vi "Single Channel_stepper.vi"(4 "B":bool, 5 "A":bool, 6 "DIR":bool, 7 "Period (Ticks)":u32=2000, 8 "STBY":bool, 9 "ENA":bool, 10 "Duty":fxp<+,32,0>, 11 "I/O Channel":T1={"Encoder C"="ConnectorA/DIO13", "Encoder B"="ConnectorA/DIO12", "Encoder A"="ConnectorA/DIO11", "PWM"="ConnectorA/DIO10", "DIR"="ConnectorA/DIO9", "STBY"="ConnectorA/DIO8", "ENA"="ConnectorA/DIO7"}) -> (1 "C":bool)   [LabVIEW 2018]
uses:
  <vilib>/rvi/eio/common/nirviEmuTemplateMethod_errors.vi
  <vilib>/eio/EIONode/EIONode.xnode
  jmslib.lvlib
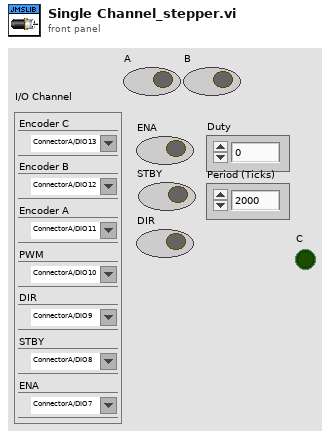
[diagram p1: front panel]
types:
  T1 = cluster{"Encoder C":refnum<k21>, "Encoder B":refnum<k21>, "Encoder A":refnum<k21>, "PWM":refnum<k21>, "DIR":refnum<k21>, "STBY":refnum<k21>, "ENA":refnum<k21>}
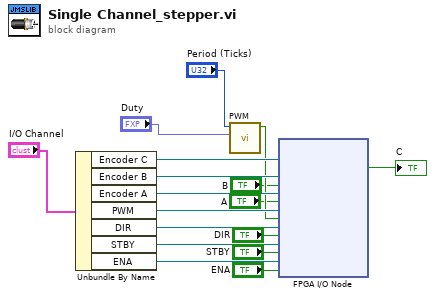
[diagram p0: block diagram]
diagram:
  n1 = Unbundle By Name("I/O Channel") -> ("Encoder C"=w16:refnum<k21>, "Encoder B"=w15:refnum<k21>, "Encoder A"=w14:refnum<k21>, "PWM"=w13:refnum<k21>, "DIR"=w12:refnum<k21>, "STBY"=w11:refnum<k21>, "ENA"=w10:refnum<k21>)
  n2 = call "PWM.vi"("Duty Cycle"="Duty", "Period (Ticks)"="Period (Ticks)") -> ("PWM Out"=w5:bool)  [unwired: 8 in, 1 out]
  n3 = xnode "FPGA I/O Node"("FPGA I/O In"=w16, "I/O Item"="B", "FPGA I/O In"=w15, "I/O Item"="A", "FPGA I/O In"=w14, "I/O Item"=w5, "FPGA I/O In"=w13, "I/O Item"="DIR", "FPGA I/O In"=w12, "I/O Item"="STBY", "FPGA I/O In"=w11, "I/O Item"="ENA", "FPGA I/O In"=w10) -> ("I/O Item"=→"C":bool)  [unwired: 7 out]
